vi "Initialise Panel.vi"(7 "This VI":refnum<vi>, 11 "UI Ref":T1) -> (0 "error out":errorcluster)   [LabVIEW 2021]
doc: "This vi sets up the UI panels, so it is ready to use."
uses:
  Control/User Interface Reference Cluster.ctl
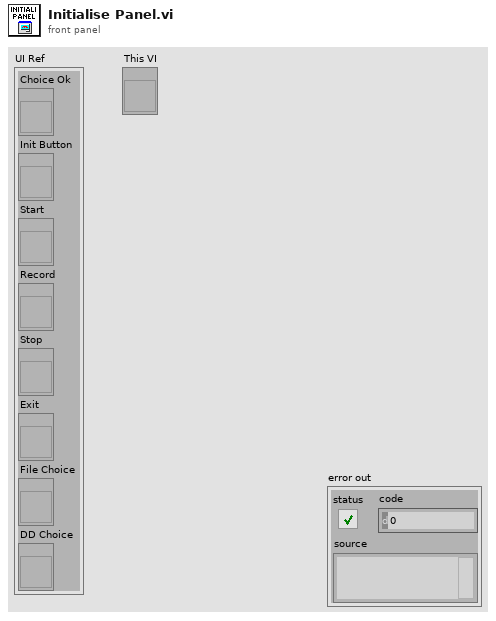
[diagram p1: front panel]
types:
  T1 = typedef "User Interface Reference Cluster.ctl" = cluster{"Choice Ok":refnum<vi>, "Init Button":refnum<vi>, "Start":refnum<vi>, "Record":refnum<vi>, "Stop":refnum<vi>, "Exit":refnum<vi>, "File Choice":refnum<vi>, "DD Choice":refnum<vi>}
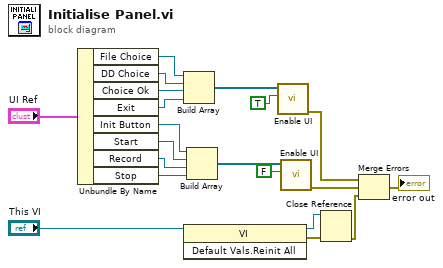
[diagram p0: block diagram]
diagram:
  n1 = Unbundle By Name("UI Ref") -> ("File Choice"=w5:refnum<vi>, "DD Choice"=w6:refnum<vi>, "Choice Ok"=w19:refnum<vi>, "Exit"=w14:refnum<vi>, "Init Button"=w13:refnum<vi>, "Start"=w10:refnum<vi>, "Record"=w11:refnum<vi>, "Stop"=w12:refnum<vi>)
  n2 = Build Array(w5, w6, w19, w14) -> (w18:refnum<vi>[])
  n3 = invoke class="VI" method="Default Vals.Reinit All"(reference="This VI") -> (reference out=w2:refnum<vi>, error out=w3:errorcluster)  [unwired: 2 in, 1 out]
  n4 = Build Array(w13, w10, w11, w12) -> (w15:refnum<vi>[])
  n5 = call "Enable UI.vi"("Enable?"=TRUE, "output cluster"=w18) -> ("error out"=w9:errorcluster)  [unwired: 9 in]
  n6 = call "Enable UI.vi"("Enable?"=FALSE, "output cluster"=w15) -> ("error out"=w8:errorcluster)  [unwired: 9 in]
  n7 = Close Reference(reference=w2, error in (no error)=w3) -> (error out=w1:errorcluster)
  n8 = Merge Errors(w9, w8, w1) -> (→"error out":errorcluster)
